vi "FeederBeam.vi"(8 "error in (no error)":errorcluster) -> (0 "error out":errorcluster)   [LabVIEW 2013]
doc: "Use this template to build a VI to use as a subVI."
uses:
  704IO.dll
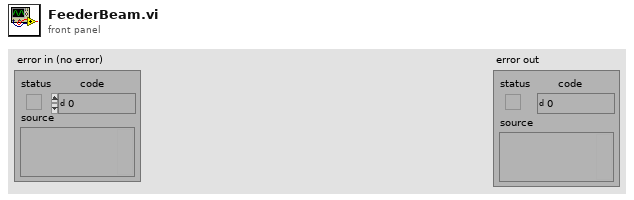
[diagram p1: front panel]
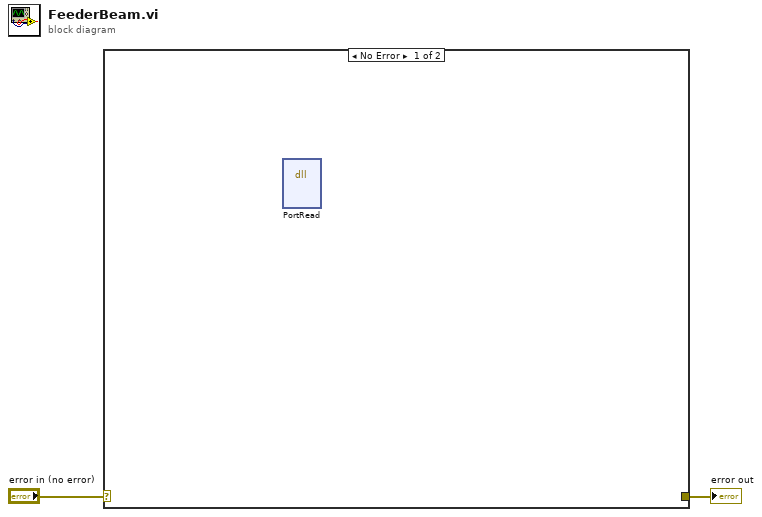
[diagram p0: block diagram]
diagram:
  n1 = case shown="No Error" "error in (no error)" {
    selector: "error in (no error)" -> [_ w3]
    tunnel: [_ w3] -> w1
    frame No Error {
      n2 = dll-call lib="C:/Users/Radu Darie/Documents/GitHub/ParkinsonsCorridor/704IO.dll" fn="PortRead"() -> ()  [unwired: 10 in, 2 out]
    }
    frame Error {
    }
  }
  "error out" <- w1
